vi "grabAcquire_action.vi"(0 "HGF_ImaqFg":refnum<class "HGF_ImaqFg.lvclass">, 2 "Image In":T1, 3 "Wait for Next Buffer? (Yes)":bool=TRUE, 5 "error in (no error)":errorcluster) -> (14 "dup HGF_ImaqFg":refnum<class "HGF_ImaqFg.lvclass">, 16 "Image Out":T1, 17 "Acquired Buffer Number":u32, 19 "error out":errorcluster)   [LabVIEW 2014, in "HGF_IMAQ.lvlib" / "HGF_ImaqFg.lvclass"]
doc: "Acquires an image from a grab acquisition. Use the grab function for high-speed image acquisition.\n\nWait parameter is ignored by IMAQ for USB."
uses:
  HGF_ImaqFg.lvclass
  <vilib>/vision/Image Controls.llb/IMAQ Image.ctl
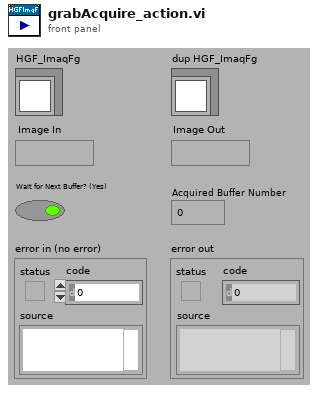
[diagram p1: front panel]
types:
  T1 = typedef "IMAQ Image.ctl" = refnum<image>
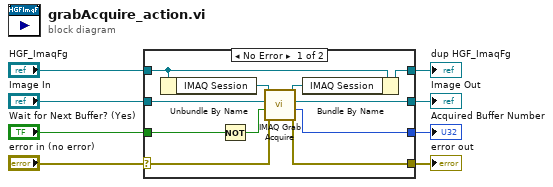
[diagram p0: block diagram]
diagram:
  n1 = case shown="No Error" "error in (no error)" {
    selector: "error in (no error)" -> [w9 w20]
    tunnel: "Image In" -> [w19 w21]
    tunnel: [w18 w21] -> w7
    tunnel: "HGF_ImaqFg" -> [w16 w22]
    tunnel: [w15 w22] -> w5
    tunnel: [w13 w20] -> w4
    tunnel: [w12 _] -> w3
    tunnel: "Wait for Next Buffer? (Yes)" -> [w11 _]
    frame No Error {
      n2 = Unbundle By Name(w16) -> ("IMAQ Session"=w17:refnum<k11>)
      n3 = Not(x=w11) -> (.not. x?=w10:bool)
      n4 = call <vilib>:"IMAQ Grab Acquire.vi"("error in (no error)"=w9, "Immediate?"=w10, "Image In"=w19, "IMAQ Session In"=w17) -> ("error out"=w13:errorcluster, "Acquired Buffer Number"=w12:u32, "Image Out"=w18:T1, "IMAQ Session Out"=w14:refnum<k11>)  [unwired: 4 out]
      n5 = Bundle By Name(cluster=w16, "IMAQ Session"=w14) -> (w15:refnum<class "HGF_ImaqFg.lvclass">)
    }
    frame Error {
    }
  }
  "error out" <- w4
  "dup HGF_ImaqFg" <- w5
  "Image Out" <- w7
  "Acquired Buffer Number" <- w3
